vi "Initialize.vi"(7 "option string":string="Simulate=0,RangeCheck=1,QueryInstrStatus=0,Cache=1", 8 "error in (no error)":errorcluster, 9 "reset device (Yes)":bool=TRUE, 10 "id query (Yes)":bool=TRUE, 11 "Keysight44xx in":refnum<class "Keysight44xx.lvclass">) -> (0 "error out":errorcluster, 3 "Keysight44xx out":refnum<class "Keysight44xx.lvclass">)   [LabVIEW 2018, in "SpecAnPlugins.lvlib" / "Keysight44xx.lvclass"]
doc: "This function opens a reference to the Spectrum Analyzer and sets the connected boolean to true."
uses:
  Keysight44xx.lvclass
  C:/Users/ico/Documents/Projects/NistPluggableModules/SpecAn/SpecAnPlugins/SpecAnBaseClass/SpecAnBase.lvclass
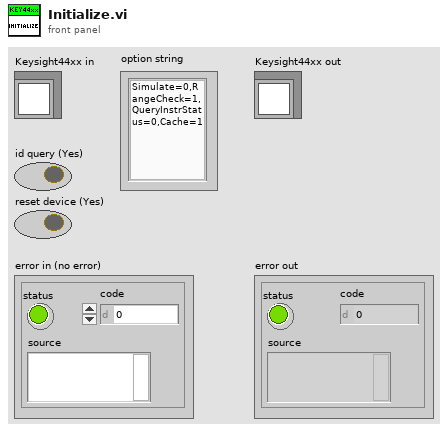
[diagram p1: front panel]
types:
  T1 = typedef "SpecAnPlugins.lvlib/SpecAnBase.lvclass/Acquisition.ctl" = cluster{"Handle":string, "Connected":bool, "Enabled":bool, "SweepModeContinuous":bool, "NumberOfSweeps":i32, "DetectorTypeAuto":bool, "DetectorType":i32, "VerticalScale":i32, "MaximumTime(seconds)":dbl}
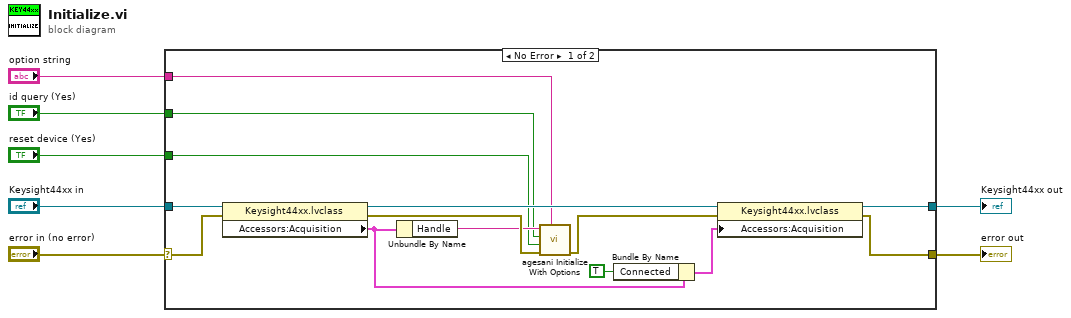
[diagram p0: block diagram]
diagram:
  n1 = case shown="No Error" "error in (no error)" {
    selector: "error in (no error)" -> [w20 w23]
    tunnel: [w17 w23] -> w6
    tunnel: "Keysight44xx in" -> [w21 w22]
    tunnel: [w16 w22] -> w4
    tunnel: "option string" -> [w11 _]
    tunnel: "id query (Yes)" -> [w10 _]
    tunnel: "reset device (Yes)" -> [w9 _]
    frame No Error {
      n2 = property class="Keysight44xx.lvclass"(reference=w21, error in=w20) -> (reference out=w15:refnum<class "Keysight44xx.lvclass">, error out=w19:errorcluster, "Accessors:Acquisition"=w14:T1)
      n3 = Unbundle By Name(w14) -> ("Handle"=w12:string)
      n4 = call <instrlib>:"agesani Initialize With Options.vi"("option string (\"Simulate=0,RangeCheck=1,QueryInstrStatus=0,Cache=1\")"=w11, "error in (no error)"=w19, "reset device (Yes)"=w9, "id query (Yes)"=w10, "resource name"=w12) -> ("error out"=w18:errorcluster)  [unwired: 5 in, 1 out]
      n5 = Bundle By Name(cluster=w14, "Connected"=TRUE) -> (w13:T1)
      n6 = property class="Keysight44xx.lvclass"(reference=w15, error in=w18, "Accessors:Acquisition"=w13) -> (reference out=w16:refnum<class "Keysight44xx.lvclass">, error out=w17:errorcluster)
    }
    frame Error {
    }
  }
  "error out" <- w6
  "Keysight44xx out" <- w4
